vi "Auton Builder.vi"() -> ()   [LabVIEW 2018]
uses:
  Typedef/Robot Settings.ctl
  Typedef/Data Point.ctl
  Typedef/Robot Starting Position.ctl
  Typedef/Sequence Command.ctl
  Typedef/Plate Arrangement.ctl
  <vilib>/Utility/miscctls.llb/LVRowAndColumnTypeDef.ctl
panel:
  in  "Start Position Names":T1
  in  "Stop?":bool
  in  "Tab Control":enum32{"Builder", "Raw Sequence", "Settings"}(tab)
  in  "Start Position":T1
  in  "Reverse Path":bool
  in  "Data Points":T2[](array[typedef])=[{"X"=68.0, "Y"=162.0, "Theta"=0.0, "Speed %"=0.0, "Disabled?"=FALSE}]
  in  "Open":bool
  in  "Save":bool
  in  "Reset":bool
  in  "Send to Robot":bool
  in  "Simulate":bool
  in  "Name":string
  out "Field Half":cluster{dbl[], dbl[]}[](graph)=[{[48.5, 82.0, 82.0, 48.5, 48.5], [176.25, 176.25, 147.75, 147.75, 176.25]}, {[68.0], [162.0]}, {[68.0], [162.0]}, {[81.13940299900052], [156.48469503745656]}, {[54.86059700099948], [167.51530496254344]}]
  in  "Cancel":bool
  out "Location Names":string[](array[string])=["Center", "Left Level 1", "Right Level 1", "Left Level 2", "Right Level 2"]
  in  "Locations":cluster{"X":dbl, "Y":dbl}[](array[cluster])=[{"X"=68.0, "Y"=162.0}, {"X"=68.0, "Y"=212.0}, {"X"=68.0, "Y"=112.0}, {"X"=19.5, "Y"=212.0}, {"X"=19.5, "Y"=112.0}]
  in  "Path Folder":path=path "C:/Users/RoboChargers/Documents/LabVIEW Data/Deep-Space-2019/Auton/Paths"
  in  "Robot Settings":T3={"Width"=28.5, "Length"=33.5, "Center of Rotation"=19.5} caption="Robot Settings w/ Bumpers"
  # "LEFT"
  # "FAR"
  # "NEAR"
  # "RIGHT"
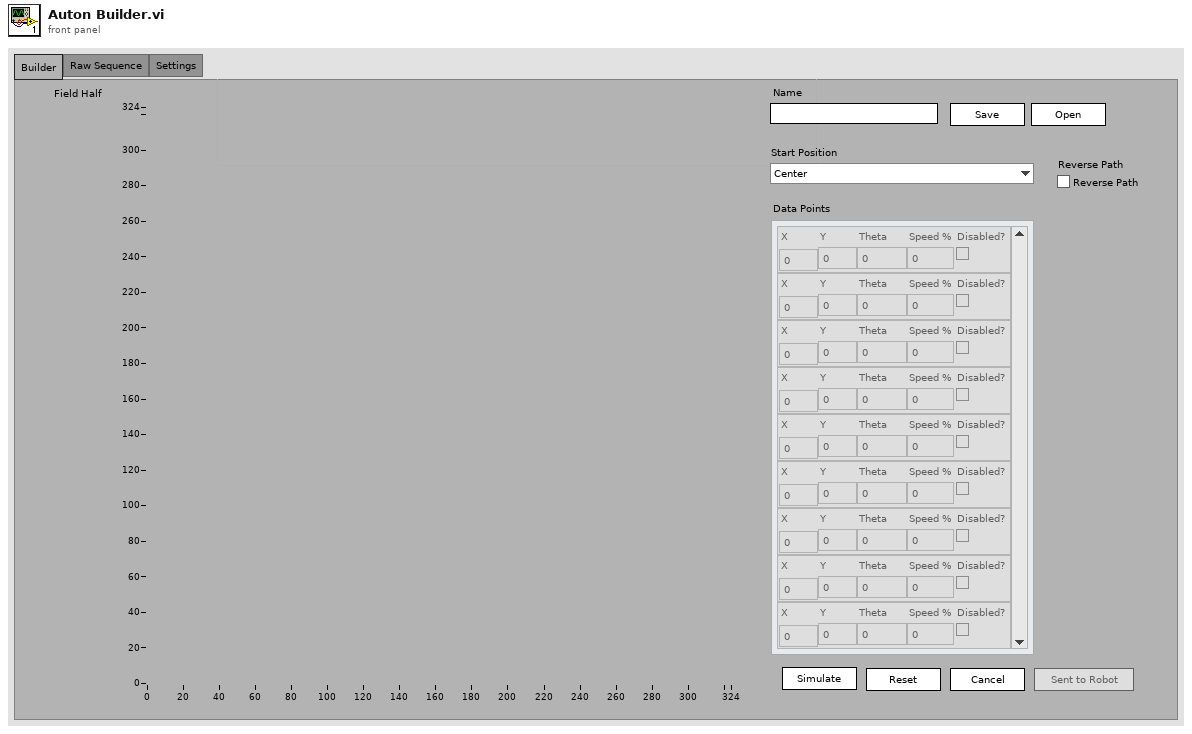
[diagram p1: front panel]
types:
  T1 = typedef "Robot Starting Position.ctl" = enum16{"Center", "Left Level 1", "Right Level 1", "Left Level 2", "Right Level 2"}
  T2 = typedef "Data Point.ctl" = cluster{"X":dbl, "Y":dbl, "Theta":dbl, "Speed %":dbl, "Disabled?":bool}
  T3 = typedef "Robot Settings.ctl" = cluster{"Width":dbl, "Length":dbl, "Center of Rotation":dbl}
  T4 = typedef "Sequence Command.ctl" = cluster{"Sequence Name":string, "Plate Arrangement":T5, "Command Name":string, "Data":variant, "Sequence Number":u32}
  T5 = typedef "Plate Arrangement.ctl" = cluster{"LR*":bool, "LL*":bool, "RL*":bool, "RR*":bool}
  T6 = typedef "LVRowAndColumnTypeDef.ctl" = cluster{"Row":i32, "Column":i32}
  T7 = cluster{"Field Half":cluster{dbl[], dbl[]}[], "Current Command":T4, "Robot Position":cluster{"x":dbl, "y":dbl}, "Theta":dbl, "y position":dbl, "Active Cell":T6, "Robot Index":i32, "Sequence OK?":bool, "Start Position":cluster{"x":dbl, "y":dbl}, "Field Selection":string, "Simulation Index":i32, "Sim Robot Index":i32, "Active Path":path, "Load Index":i32, "Graph Index":i32, "Data Points Index":i32, "Data Points":T2[], "Path Index":i32, "Path L Index":i32, "Path R Index":i32}
  T8 = typedef "LVPoint32TypeDef.ctl" = cluster{"Horizontal":i32, "Vertical":i32}
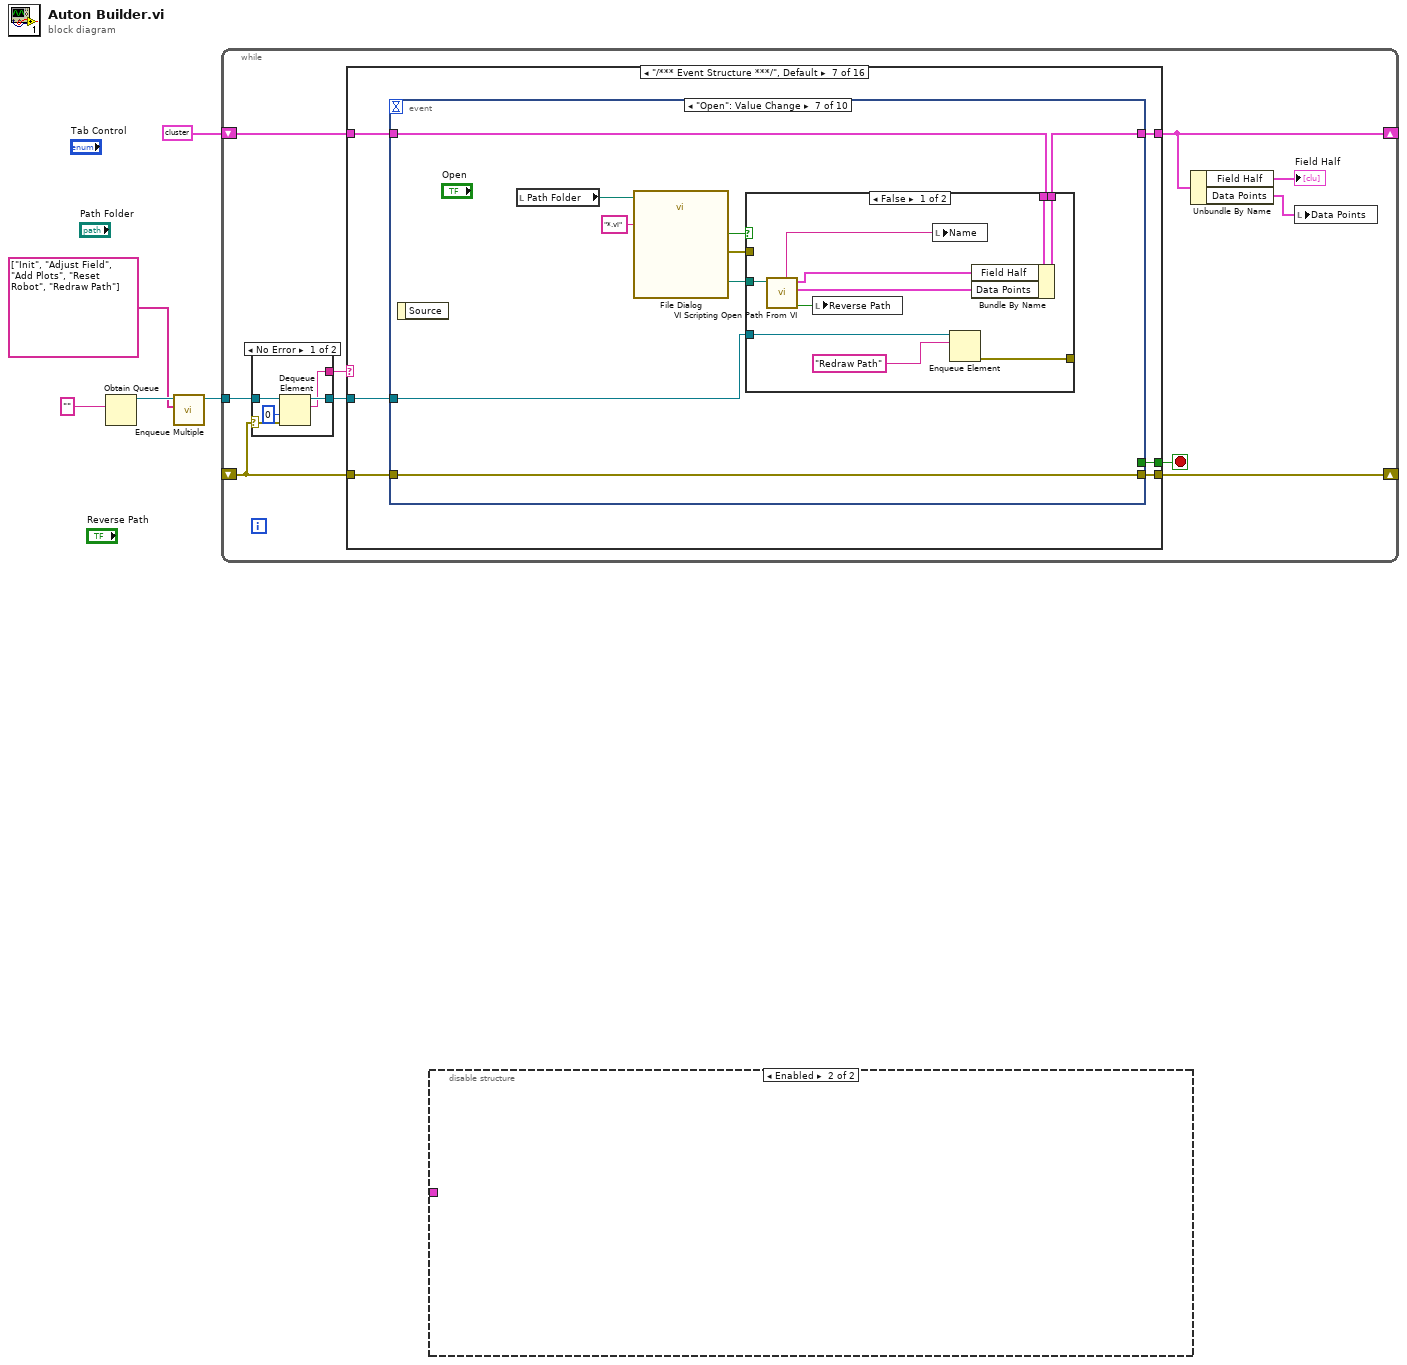
[diagram p0: block diagram]
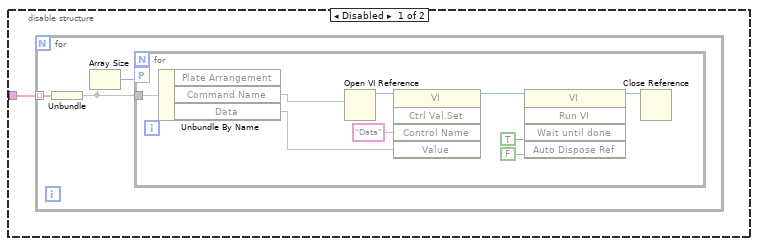
[diagram p2: hidden frame]
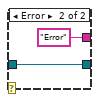
[diagram p3: hidden frame]
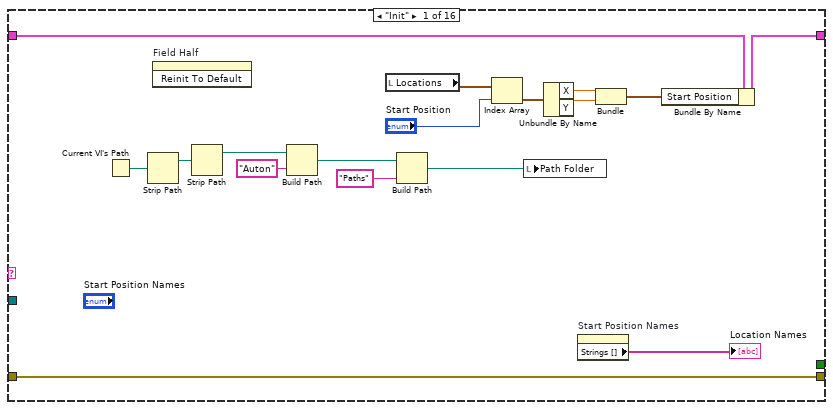
[diagram p4: hidden frame]
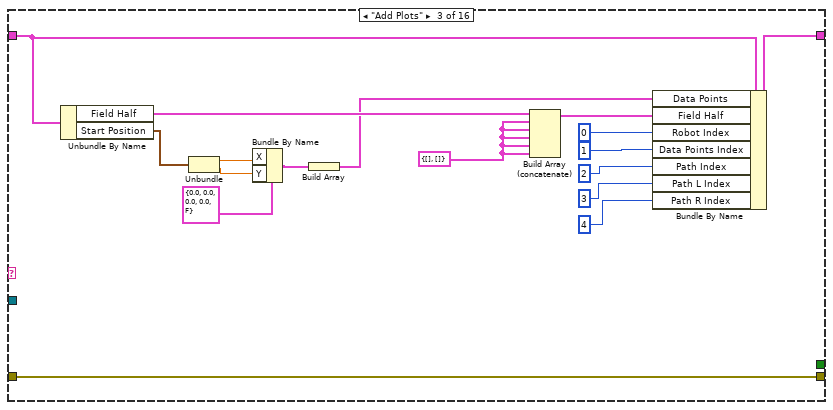
[diagram p6: hidden frame]
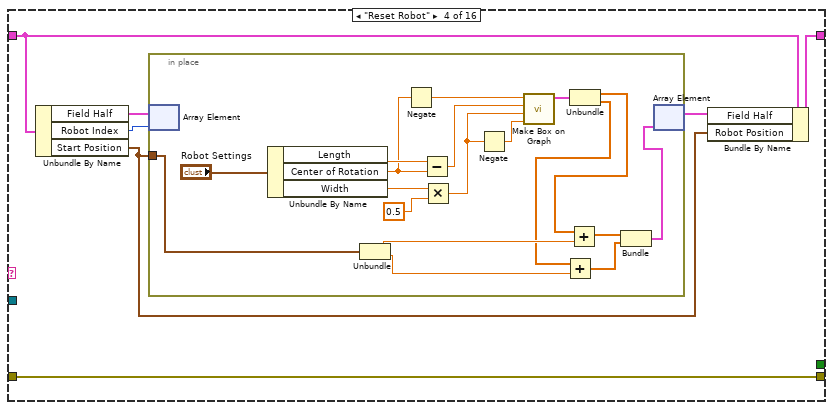
[diagram p7: hidden frame]
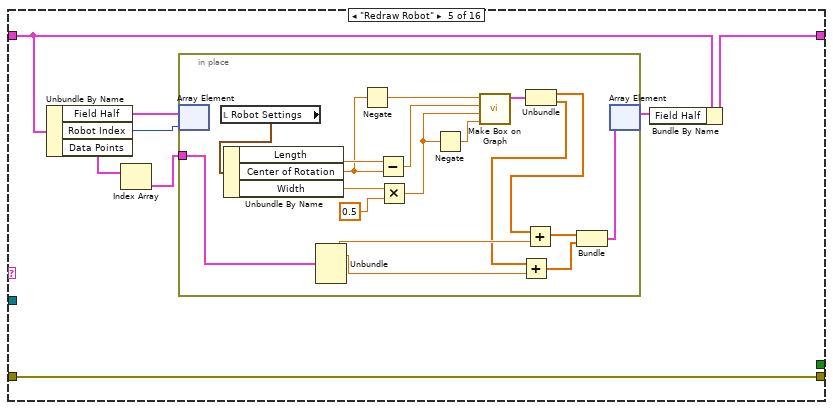
[diagram p8: hidden frame]
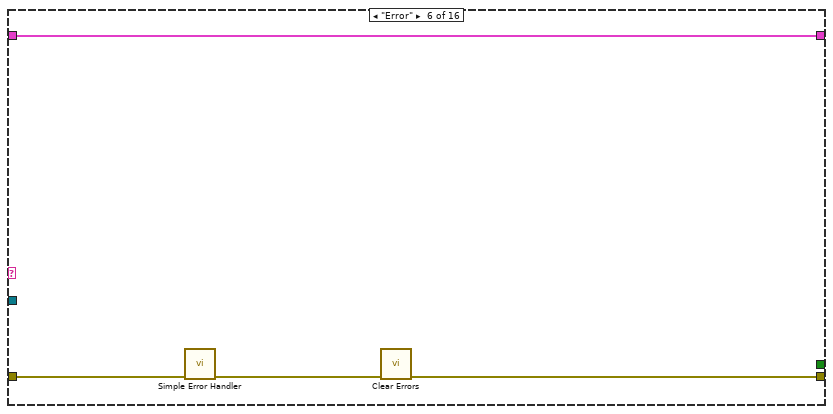
[diagram p9: hidden frame]
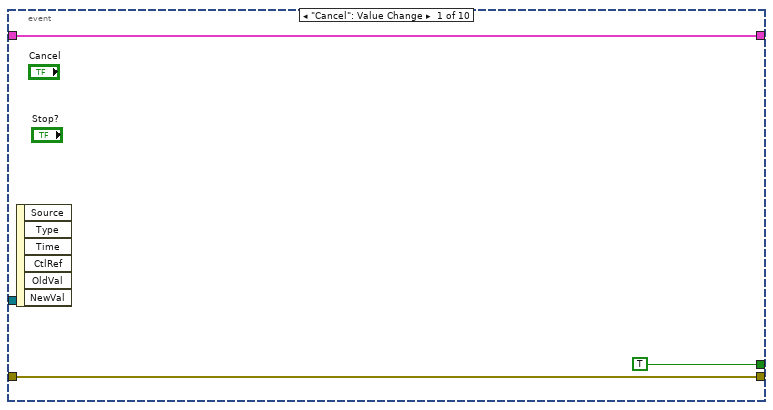
[diagram p10: hidden frame]
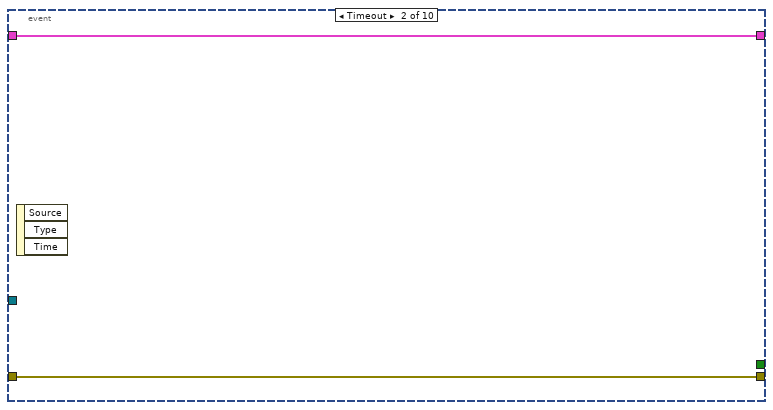
[diagram p11: hidden frame]
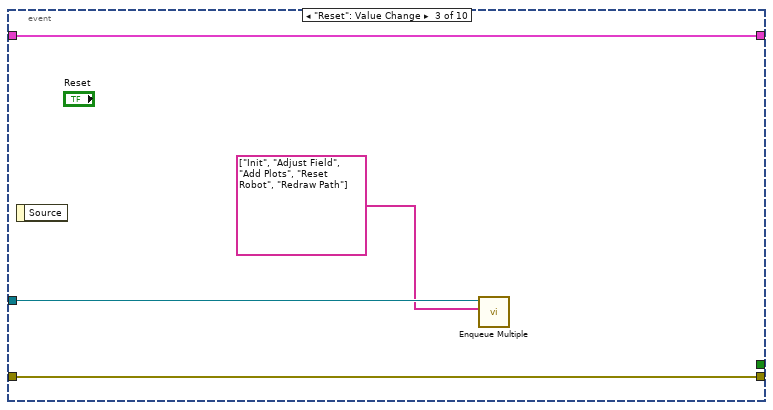
[diagram p12: hidden frame]
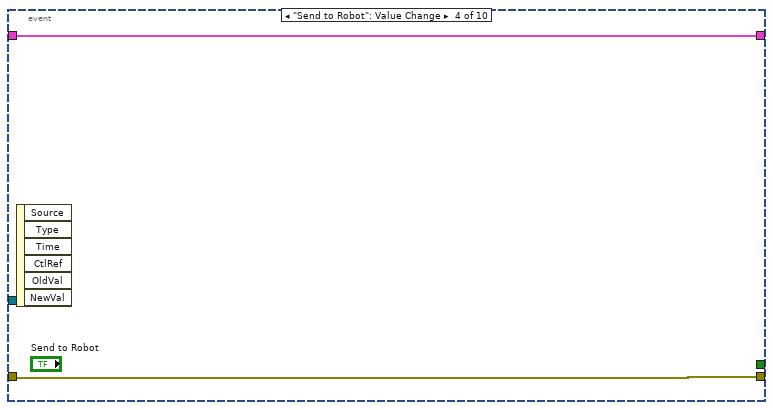
[diagram p13: hidden frame]
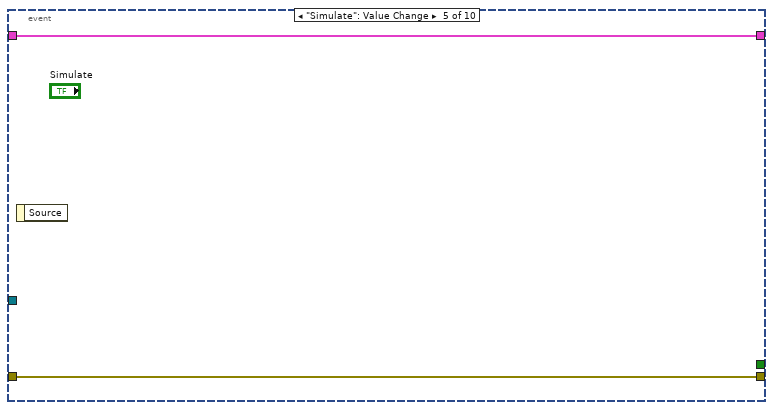
[diagram p14: hidden frame]
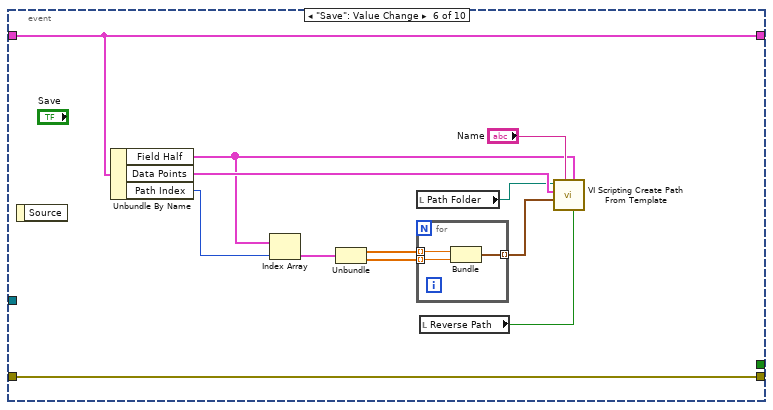
[diagram p15: hidden frame]
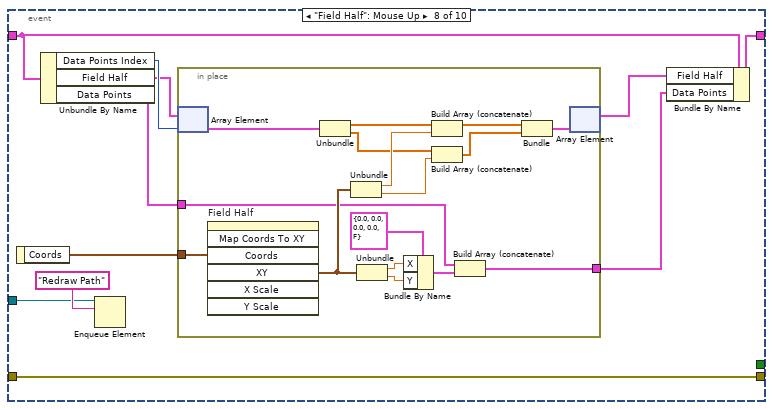
[diagram p17: hidden frame]
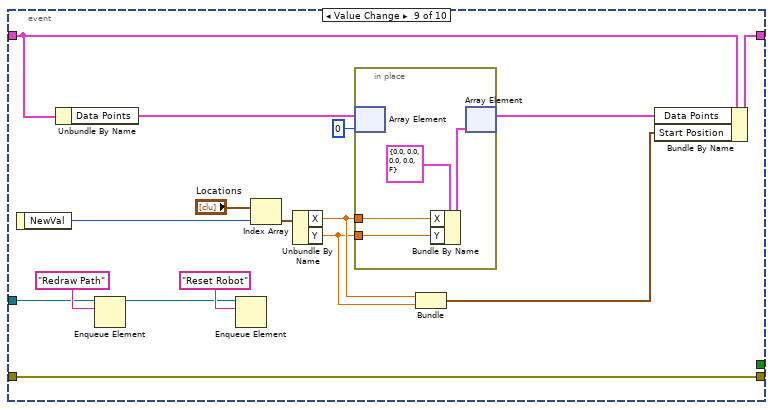
[diagram p18: hidden frame]
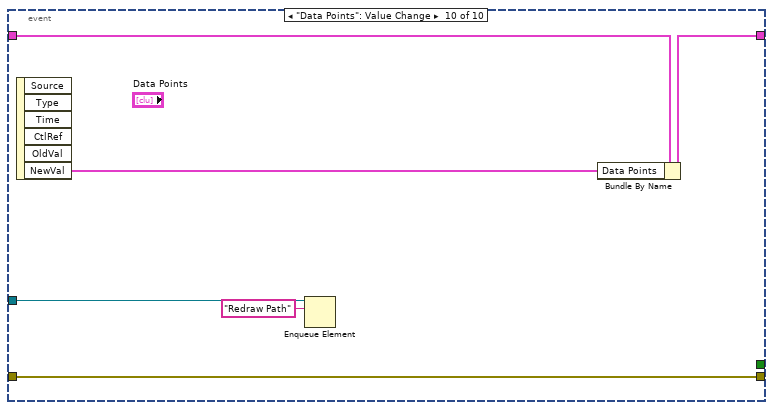
[diagram p19: hidden frame]
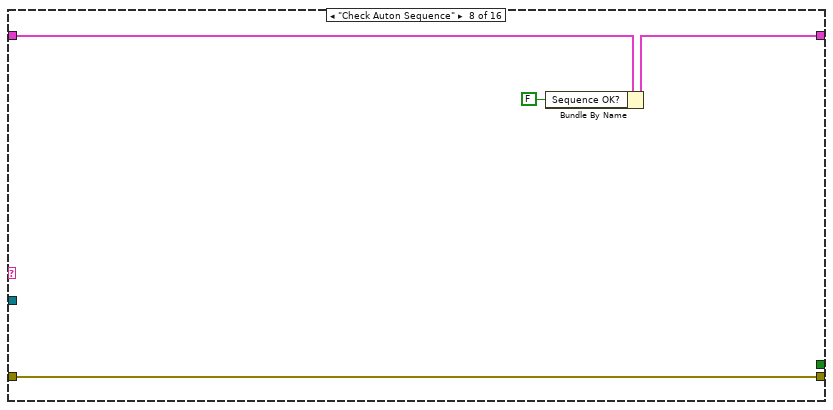
[diagram p20: hidden frame]
diagram:
  n1 = Obtain Queue(element data type="") -> (queue out=w4:refnum<queue>)  [unwired: 4 in, 2 out]
  n2 = call "Enqueue Multiple.vi"("Array"=string[] ["Init", "Adjust Field", "Add Plots", "Reset Robot", "Redraw Path"], "Queue in"=w4) -> ("Queue out"=w3:refnum<queue>)  [unwired: 8 in, 1 out]
  n3 = while {
    shift-right: [w9] -> _
    shift-left: T7 {"Field Half"=[], "Current Command"={"Sequence Name"="", "Plate Arrangement"={"LR*"=FALSE, "LL*"=FALSE, "RL*"=FALSE, "RR*"=FALSE}, "Command Name"="", "Data"=variant, "Sequence Number"=0}, "Robot Position"={"x"=0.0, "y"=0.0}, "Theta"=0.0, "y position"=0.0, "Active Cell"={"Row"=0, "Column"=0}, "Robot Index"=0, "Sequence OK?"=FALSE, "Start Position"={"x"=0.0, "y"=0.0}, "Field Selection"="", "Simulation Index"=0, "Sim Robot Index"=0, "Active Path"=path "", "Load Index"=0, "Graph Index"=0, "Data Points Index"=0, "Data Points"=[], "Path Index"=0, "Path L Index"=0, "Path R Index"=0} ("output cluster") -> [w15]
    shift-right: [w11] -> _
    shift-left: _ -> [w10]
    tunnel: w3 -> [w14]
    stop <- w7 stop-if-true
    n4 = case shown="No Error" w10 {
      selector: w10 -> [w18 _]
      tunnel: w14 -> [w20 w22]
      tunnel: [w19 w22] -> w13
      tunnel: [w17 "Error"] -> w12
      frame No Error {
        n5 = Dequeue Element(queue=w20, timeout in ms (-1)=0, error in (no error)=w18) -> (queue out=w19:refnum<queue>, element=w17:string)  [unwired: 2 out]
      }
      frame Error {
      }
    }
    n6 = case shown="\"/*** Event Structure ***/\", Default" w12 {
      tunnel: [_ _ _ _ _ _ w119 _ _ _ _ _ _ _ _ _] -> w7
      tunnel: w15 -> [w39 w40 w56 w64 w90 w113 w118 w223 w235 w250 w262 w278 w307 w312 w314 w316]
      tunnel: [w38 w40 w58 w65 w91 w113 w117 w222 w228 w246 w261 w276 w307 w310 w314 w316] -> w9
      tunnel: w13 -> [_ _ _ _ _ _ w116 _ _ _ _ w269 _ _ _ _]
      tunnel: [w37 w41 w54 w63 w89 w112 w114 w224 w226 w244 w263 w279 w306 w311 w313 w315] -> w11
      tunnel: w10 -> [w37 w41 w54 w63 w89 w111 w115 w224 w226 w244 w263 w279 w306 w311 w313 w315]
      frame "Init" {
        n7 = Current VI's Path() -> (path=w36:path)
        n8 = Strip Path(path=w36) -> (stripped path=w35:path)  [unwired: 1 out]
        n9 = invoke on="Field Half" class="XYGraph (strict)" method="Reinit To Default"() -> ()  [unwired: 3 in, 3 out]
        n10 = Strip Path(path=w35) -> (stripped path=w34:path)  [unwired: 1 out]
        n11 = Build Path(base path=w34, name or relative path="Auton") -> (appended path=w32:path)
        n12 = local read "Locations"() -> (w24:cluster{"X":dbl, "Y":dbl}[])
        n13 = Build Path(base path=w32, name or relative path="Paths") -> (appended path=w30:path)
        n14 = Index Array(array=w24, index="Start Position") -> (element=w28:cluster{"X":dbl, "Y":dbl})
        n15 = local write "Path Folder"(w30) -> ()
        n16 = Unbundle By Name(w28) -> ("X"=w27:dbl, "Y"=w26:dbl)
        n17 = property on="Start Position Names" class="Enum (strict)"() -> ("Strings []"=→"Location Names":string[])  [unwired: 2 in, 2 out]
        n18 = Bundle("X"=w27, "Y"=w26) -> (w25:cluster{"X":dbl, "Y":dbl})  [unwired: 1 in]
        n19 = Bundle By Name(cluster=w39, "Start Position"=w25) -> (w38:T7)
      }
      frame "Adjust Field" {
      }
      frame "Add Plots" {
        w47 = cluster{dbl[], dbl[]} {[], []} ("element")
        n20 = Unbundle By Name(w56) -> ("Field Half"=w55:cluster{dbl[], dbl[]}[], "Start Position"=w48:cluster{"x":dbl, "y":dbl})
        n21 = Unbundle(w48) -> ("x"=w45:dbl, "y"=w44:dbl)
        n22 = Bundle By Name(cluster=T2 {"X"=0.0, "Y"=0.0, "Theta"=0.0, "Speed %"=0.0, "Disabled?"=FALSE} ("Cluster"), "X"=w45, "Y"=w44) -> (w43:T2)
        n23 = Build Array(w43) -> (w42:T2[])
        n24 = Build Array (concatenate)(w55, w47, w47, w47, w47, w47) -> (w57:cluster{dbl[], dbl[]}[])
        n25 = Bundle By Name(cluster=w56, "Data Points"=w42, "Field Half"=w57, "Robot Index"=0, "Data Points Index"=1 ("Spline Index"), "Path Index"=2 ("Spline Index"), "Path L Index"=3 ("Spline Index"), "Path R Index"=4 ("Spline Index")) -> (w58:T7)
      }
      frame "Reset Robot" {
        n26 = Unbundle By Name(w64) -> ("Field Half"=w62:cluster{dbl[], dbl[]}[], "Robot Index"=w61:i32, "Start Position"=w59:cluster{"x":dbl, "y":dbl})
        n27 = in-place {
          in-place-border: w59 -> [w83]
          n28 = in-place-array #1(w62, w61) -> ()  [unwired: 1 out]
          n29 = Unbundle By Name("Robot Settings") -> ("Length"=w73:dbl, "Center of Rotation"=w72:dbl, "Width"=w77:dbl)
          n30 = Unbundle(w83) -> ("x"=w82:dbl, "y"=w81:dbl)
          n31 = Negate(x=w72) -> (-x=w74:dbl)
          n32 = Subtract(x=w73, y=w72) -> (x-y=w71:dbl)
          n33 = Multiply(x=w77, y=0.5 ("x")) -> (x*y=w76:dbl)
          n34 = Negate(x=w76) -> (-x=w75:dbl)
          n35 = call "Make Box on Graph.vi"("Y2"=w75, "Y1"=w76, "X2"=w71, "X1"=w74) -> ("Output Graph"=w69:cluster{dbl[], dbl[]})  [unwired: 7 in]
          n36 = Unbundle(w69) -> (w68:dbl[], w67:dbl[])
          n37 = Add(x=w67, y=w81) -> (x+y=w80:dbl[])
          n38 = Add(x=w68, y=w82) -> (x+y=w79:dbl[])
          n39 = Bundle(w79, w80) -> (w66:cluster{dbl[], dbl[]})  [unwired: 1 in]
          n40 = in-place-array #1(w66) -> (w60:cluster{dbl[], dbl[]}[])  [unwired: 1 out]
        }
        n41 = Bundle By Name(cluster=w64, "Field Half"=w60, "Robot Position"=w59) -> (w65:T7)
      }
      frame "Redraw Robot" {
        n42 = Unbundle By Name(w90) -> ("Field Half"=w88:cluster{dbl[], dbl[]}[], "Robot Index"=w87:i32, "Data Points"=w86:T2[])
        n43 = Index Array(array=w86) -> (element=w85:T2)  [unwired: 1 in]
        n44 = in-place {
          in-place-border: w85 -> [w109]
          n45 = in-place-array #2(w88, w87) -> ()  [unwired: 1 out]
          n46 = local read "Robot Settings"() -> (w93:T3)
          n47 = Unbundle By Name(w93) -> ("Length"=w100:dbl, "Center of Rotation"=w99:dbl, "Width"=w104:dbl)
          n48 = Unbundle(w109) -> ("X"=w108:dbl, "Y"=w107:dbl)  [unwired: 3 out]
          n49 = Negate(x=w99) -> (-x=w101:dbl)
          n50 = Subtract(x=w100, y=w99) -> (x-y=w98:dbl)
          n51 = Multiply(x=w104, y=0.5 ("x")) -> (x*y=w103:dbl)
          n52 = Negate(x=w103) -> (-x=w102:dbl)
          n53 = call "Make Box on Graph.vi"("Y2"=w102, "Y1"=w103, "X2"=w98, "X1"=w101) -> ("Output Graph"=w96:cluster{dbl[], dbl[]})  [unwired: 7 in]
          n54 = Unbundle(w96) -> (w95:dbl[], w94:dbl[])
          n55 = Add(x=w94, y=w107) -> (x+y=w106:dbl[])
          n56 = Add(x=w95, y=w108) -> (x+y=w105:dbl[])
          n57 = Bundle(w105, w106) -> (w92:cluster{dbl[], dbl[]})  [unwired: 1 in]
          n58 = in-place-array #2(w92) -> (w84:cluster{dbl[], dbl[]}[])  [unwired: 1 out]
        }
        n59 = Bundle By Name(cluster=w90, "Field Half"=w84) -> (w91:T7)
      }
      frame "Error" {
        n60 = call <vilib>:"Simple Error Handler.vi"("error in (no error)"=w111) -> ("error out"=w110:errorcluster)  [unwired: 4 in, 4 out]
        n61 = call <vilib>:"Clear Errors.vi"("error in (no error)"=w110) -> ("error out"=w112:errorcluster)  [unwired: 5 in, 1 out]
      }
      frame "/*** Event Structure ***/", Default {
        n62 = event shown="[6] \"Open\": Value Change" {
          selector: _ -> [_ _ _ _ _ _ _ _ _ _]
          dyn-events: _ -> [_ _ _ _ _ _ _ _ _ _]
          timeout: _ -> [_ _ _ _ _ _ _ _ _ _]
          tunnel: [TRUE _ _ _ _ _ _ _ _ _] -> w119
          tunnel: w118 -> [w121 w124 w128 w130 w132 w144 w150 w174 w209 w219]
          tunnel: [w121 w124 w128 w130 w132 w144 w149 w172 w208 w218] -> w117
          tunnel: w116 -> [_ _ w127 _ _ _ w148 w168 w206 w216]
          tunnel: w115 -> [w120 w123 w126 w129 w131 w140 w156 w178 w210 w220]
          tunnel: [w120 w123 w126 w129 w131 w140 w156 w178 w210 w220] -> w114
          event "Cancel": Value Change {
            n63 = event-data() -> ()  [unwired: 1 in, 6 out]
          }
          event Timeout {
            n64 = event-data() -> ()  [unwired: 1 in, 3 out]
          }
          event "Reset": Value Change {
            n65 = event-data() -> ()  [unwired: 1 in, 1 out]
            n66 = call "Enqueue Multiple.vi"("Array"=string[] ["Init", "Adjust Field", "Add Plots", "Reset Robot", "Redraw Path"], "Queue in"=w127) -> ()  [unwired: 8 in, 2 out]
          }
          event "Send to Robot": Value Change {
            n67 = event-data() -> ()  [unwired: 1 in, 6 out]
          }
          event "Simulate": Value Change {
            n68 = event-data() -> ()  [unwired: 1 in, 1 out]
          }
          event "Save": Value Change {
            n69 = event-data() -> ()  [unwired: 1 in, 1 out]
            n70 = Unbundle By Name(w144) -> ("Field Half"=w138:cluster{dbl[], dbl[]}[], "Data Points"=w142:T2[], "Path Index"=w137:i32)
            n71 = Index Array(array=w138, index=w137) -> (element=w136:cluster{dbl[], dbl[]})
            n72 = Unbundle(w136) -> (w134:dbl[], w135:dbl[])
            n73 = local read "Path Folder"() -> (w139:path)
            n74 = for {
              tunnel: [w147] -> w141 mode=indexing
              tunnel: w135 -> [w146] mode=indexing
              tunnel: w134 -> [w145] mode=indexing
              n75 = Bundle("x"=w145, "y"=w146) -> (w147:cluster{"x":dbl, "y":dbl})  [unwired: 1 in]
            }
            n76 = local read "Reverse Path"() -> (w133:bool)
            n77 = call "VI Scripting Create Path From Template.vi"("Reverse Path?"=w133, "Graph"=w138, "Name"="Name", "path"=w141, "Data Points"=w142, "base path"=w139) -> ()  [unwired: 6 in]
          }
          event "Open": Value Change {
            n78 = event-data() -> ()  [unwired: 1 in, 1 out]
            n79 = local read "Path Folder"() -> (w154:path)
            n80 = call "File Dialog"("start path"=w154, "pattern (all files)"="*.vi") -> ("selected path"=w155:path, "cancelled"=w153:bool, "error out"=w152:errorcluster)  [unwired: 10 in, 1 out]
            n81 = case shown="False" w153 {
              tunnel: w155 -> [w166 _]
              tunnel: w150 -> [w165 w167]
              tunnel: [w163 w167] -> w149
              tunnel: w148 -> [w160 _]
              tunnel: w152 -> [_ _]
              tunnel: [w157 _] -> _
              frame False {
                n82 = call "VI Scripting Open Path From VI.vi"("Path"=w166) -> ("Reverse Path?"=w164:bool, "Data Points"=w161:T2[], "Graph"=w162:cluster{dbl[], dbl[]}[], "Name"=w158:string)  [unwired: 6 in, 1 out]
                n83 = local write "Reverse Path"(w164) -> ()
                n84 = local write "Name"(w158) -> ()
                n85 = Enqueue Element(queue=w160, element="Redraw Path") -> (error out=w157:errorcluster)  [unwired: 2 in, 2 out]
                n86 = Bundle By Name(cluster=w165, "Field Half"=w162, "Data Points"=w161) -> (w163:T7)
              }
              frame True {
              }
            }
          }
          event "Field Half": Mouse Up {
            n87 = event-data() -> ("Coords"=w177:T8)  [unwired: 1 in]
            n88 = Unbundle By Name(w174) -> ("Data Points Index"=w176:i32, "Field Half"=w175:cluster{dbl[], dbl[]}[], "Data Points"=w170:T2[])
            n89 = Enqueue Element(queue=w168, element="Redraw Path") -> ()  [unwired: 2 in, 3 out]
            n90 = in-place {
              in-place-border: w177 -> [w186]
              in-place-border: [w180] -> w171
              in-place-border: w170 -> [w179]
              n91 = in-place-array #3(w175, w176) -> (w194:cluster{dbl[], dbl[]})
              n92 = invoke on="Field Half" class="XYGraph (strict)" method="Map Coords To XY"("Coords"=w186) -> ("XY"=w184:cluster{"X":dbl, "Y":dbl})  [unwired: 6 in, 6 out]
              n93 = Unbundle(w194) -> (w192:dbl[], w191:dbl[])
              n94 = Unbundle(w184) -> ("X"=w193:dbl, "Y"=w190:dbl)
              n95 = Unbundle(w184) -> ("X"=w183:dbl, "Y"=w182:dbl)
              n96 = Bundle By Name(cluster=T2 {"X"=0.0, "Y"=0.0, "Theta"=0.0, "Speed %"=0.0, "Disabled?"=FALSE} ("Cluster"), "X"=w183, "Y"=w182) -> (w185:T2)
              n97 = Build Array (concatenate)(w192, w193) -> (w189:dbl[])
              n98 = Build Array (concatenate)(w191, w190) -> (w188:dbl[])
              n99 = Build Array (concatenate)(w179, w185) -> (w180:T2[])
              n100 = Bundle(w189, w188) -> (w187:cluster{dbl[], dbl[]})  [unwired: 1 in]
              n101 = in-place-array #3(w187) -> (w173:cluster{dbl[], dbl[]}[])  [unwired: 1 out]
            }
            n102 = Bundle By Name(cluster=w174, "Field Half"=w173, "Data Points"=w171) -> (w172:T7)
          }
          event Value Change {
            n103 = event-data() -> ("NewVal"=w200:T1)  [unwired: 1 in]
            n104 = Unbundle By Name(w209) -> ("Data Points"=w204:T2[])
            n105 = Enqueue Element(queue=w206, element="Redraw Path") -> (queue out=w198:refnum<queue>)  [unwired: 2 in, 2 out]
            n106 = Enqueue Element(queue=w198, element="Reset Robot") -> ()  [unwired: 2 in, 3 out]
            n107 = Index Array(array="Locations", index=w200) -> (element=w201:cluster{"X":dbl, "Y":dbl})
            n108 = Unbundle By Name(w201) -> ("X"=w197:dbl, "Y"=w196:dbl)
            n109 = in-place {
              in-place-border: w197 -> [w212]
              in-place-border: w196 -> [w211]
              n110 = in-place-array #4(w204, 0) -> ()  [unwired: 1 out]
              n111 = Bundle By Name(cluster=T2 {"X"=0.0, "Y"=0.0, "Theta"=0.0, "Speed %"=0.0, "Disabled?"=FALSE} ("element"), "X"=w212, "Y"=w211) -> (w214:T2)
              n112 = in-place-array #4(w214) -> (w205:T2[])  [unwired: 1 out]
            }
            n113 = Bundle("X"=w197, "Y"=w196) -> (w195:cluster{"X":dbl, "Y":dbl})  [unwired: 1 in]
            n114 = Bundle By Name(cluster=w209, "Data Points"=w205, "Start Position"=w195) -> (w208:T7)
          }
          event "Data Points": Value Change {
            n115 = event-data() -> ("NewVal"=w217:T2[])  [unwired: 1 in, 5 out]
            n116 = Enqueue Element(queue=w216, element="Redraw Path") -> ()  [unwired: 2 in, 3 out]
            n117 = Bundle By Name(cluster=w219, "Data Points"=w217) -> (w218:T7)
          }
        }
      }
      frame "Check Auton Sequence" {
        n118 = Bundle By Name(cluster=w223, "Sequence OK?"=FALSE) -> (w222:T7)
      }
      frame "Handle Graph Delete" {
        n119 = Unbundle By Name(w235) -> ("Field Half"=w229:cluster{dbl[], dbl[]}[], "Current Command"=w234:T4)
        n120 = Unbundle By Name(w234) -> ("Data"=w233:variant)
        n121 = Get Variant Attribute(Variant=w233, name="_graphIndex", default value (empty Variant)=0) -> (found=w225:bool, value=w231:i32)  [unwired: 1 in, 2 out]
        n122 = case shown="True" w225 {
          tunnel: w231 -> [_ w239]
          tunnel: w229 -> [w236 w238]
          tunnel: [w236 w237] -> w227
          frame False {
          }
          frame True {
            n123 = in-place {
              n124 = in-place-array #5(w238, w239) -> ()  [unwired: 1 out]
              n125 = in-place-array #5(cluster{dbl[], dbl[]} {[], []} ("element")) -> (w237:cluster{dbl[], dbl[]}[])  [unwired: 1 out]
            }
          }
        }
        n126 = Bundle By Name(cluster=w235, "Field Half"=w227) -> (w228:T7)
      }
      frame "Add Robot Plot" {
        n127 = Unbundle By Name(w250) -> ("Field Half"=w243:cluster{dbl[], dbl[]}[], "Current Command.Data"=w249:variant)
        n128 = Index Array(array=w243) -> (element=w241:cluster{dbl[], dbl[]})  [unwired: 1 in]
        n129 = Get Variant Attribute(Variant=w249, name="_graphPlot") -> (found=w247:bool, value=w242:variant)  [unwired: 2 in, 2 out]
        n130 = case shown="True" w247 {
          tunnel: [w251 w256] -> w245
          tunnel: w243 -> [w251 w255]
          tunnel: w242 -> [_ w254]
          tunnel: w241 -> [_ w253]
          frame False {
          }
          frame True {
            n131 = Variant To Data(type=w253, Variant=w254) -> (data=w252:cluster{dbl[], dbl[]})  [unwired: 1 in, 1 out]
            n132 = Build Array (concatenate)(w255, w252) -> (w256:cluster{dbl[], dbl[]}[])
          }
        }
        n133 = Bundle By Name(cluster=w250, "Field Half"=w245) -> (w246:T7)
      }
      frame "Update Graph Index" {
        n134 = Unbundle By Name(w262) -> ("Field Half"=w260:cluster{dbl[], dbl[]}[], "Graph Index"=w259:i32, "Current Command.Data"=w258:variant)
        n135 = in-place {
          in-place-border: w258 -> [w266]
          n136 = in-place-array #6(w260, w259) -> ()  [unwired: 1 out]
          n137 = Get Variant Attribute(Variant=w266, name="_graphPlot", default value (empty Variant)=cluster{dbl[], dbl[]} {[], []} ("value")) -> (value=w264:cluster{dbl[], dbl[]})  [unwired: 1 in, 3 out]
          n138 = in-place-array #6(w264) -> (w257:cluster{dbl[], dbl[]}[])  [unwired: 1 out]
        }
        n139 = Bundle By Name(cluster=w262, "Field Half"=w257) -> (w261:T7)
      }
      frame "Redraw Path" {
        n140 = Unbundle By Name(w278) -> ("Data Points"=w274:T2[], "Field Half"=w277:cluster{dbl[], dbl[]}[], "Data Points Index"=w270:i32, "Path Index"=w271:i32, "Path L Index"=w272:i32, "Path R Index"=w273:i32)
        n141 = Enqueue Element(queue=w269, element="Redraw Robot") -> ()  [unwired: 2 in, 3 out]
        n142 = in-place {
          in-place-border: w274 -> [w288]
          n143 = in-place-array #7(w277, w270, w271, w272, w273) -> ()  [unwired: 4 out]
          n144 = for {
            tunnel: [w305] -> w293 mode=indexing
            tunnel: w288 -> [w304] mode=indexing
            tunnel: [w303] -> w284 mode=indexing
            tunnel: [w302] -> w283 mode=indexing
            n145 = Unbundle(w304) -> ("X"=w303:dbl, "Y"=w302:dbl)  [unwired: 3 out]
            n146 = Bundle("X"=w303, "Y"=w302) -> (w305:cluster{"X":dbl, "Y":dbl})  [unwired: 1 in]
          }
          n147 = local read "Robot Settings"() -> (w281:T3)
          n148 = call "Path Inject Points.vi"("Distance"=1.0, "Path"=w293) -> ("Path out"=w298:cluster{dbl, dbl}[])  [unwired: 9 in]
          n149 = Bundle(w284, w283) -> (w282:cluster{dbl[], dbl[]})  [unwired: 1 in]
          n150 = Unbundle By Name(w281) -> ("Width"=w280:dbl)
          n151 = call "Path Smoother.vi"("tolerance"=0.001, "B"=0.95, "A"=0.05, "Path"=w298) -> ("SmoothPath"=w292:cluster{dbl, dbl}[])  [unwired: 7 in]
          n152 = for {
            tunnel: w292 -> [w301] mode=indexing
            tunnel: [w300] -> w290 mode=indexing
            tunnel: [w299] -> w291 mode=indexing
            n153 = Unbundle(w301) -> (w300:dbl, w299:dbl)
          }
          n154 = Bundle(w290, w291) -> (w285:cluster{dbl[], dbl[]})  [unwired: 1 in]
          n155 = call "Path to Wheel Path.vi"("Wheelbase (in)"=w280, "waypoints"=w285) -> ("out"=w289:cluster{dbl[], dbl[]}[])  [unwired: 9 in]
          n156 = Index Array(array=w289) -> (element #1=w286:cluster{dbl[], dbl[]}, element #2=w287:cluster{dbl[], dbl[]})  [unwired: 2 in]
          n157 = in-place-array #7(w282, w285, w286, w287) -> (w275:cluster{dbl[], dbl[]}[])  [unwired: 4 out]
        }
        n158 = Bundle By Name(cluster=w278, "Field Half"=w275) -> (w276:T7)
      }
      frame "/**** Simulation Functions ****/" {
      }
      frame "Simulation Init" {
        n159 = Bundle By Name(cluster=w312, "Simulation Index"=0, "Sim Robot Index"=0) -> (w310:T7)
      }
      frame "Select Field String" {
      }
      frame "/**** File Operations ****/" {
      }
    }
    n160 = Unbundle By Name(w9) -> ("Field Half"=→"Field Half":cluster{dbl[], dbl[]}[], "Data Points"=w6:T2[])
    n161 = local write "Data Points"(w6) -> ()
  }
  n162 = disable-structure shown="Enabled" {
    disable-tunnel: _ -> [w317 _]
    frame Disabled {
      n163 = for {
        tunnel: w317 -> [w320] mode=indexing
        n164 = Unbundle(w320) -> ("Sequence Array"=w318)
        n165 = Array Size(array=w318) -> (size(s)=w319:i32)
        n166 = for {
          tunnel: w318 -> [w329]
          workers-P: w319 -> [_]
          n167 = Unbundle By Name(w329) -> ("Command Name"=w325, "Data"=w327)  [unwired: 1 out]
          n168 = Open VI Reference(vi path=w325) -> (vi reference=w328:refnum<vi>)  [unwired: 5 in, 1 out]
          n169 = invoke class="VI" method="Ctrl Val.Set"(reference=w328, "Control Name"="Data", "Value"=w327) -> (reference out=w324:refnum<vi>)  [unwired: 2 in, 4 out]
          n170 = invoke class="VI" method="Run VI"(reference=w324, "Wait until done"=TRUE ("Wait Until Done"), "Auto Dispose Ref"=FALSE ("Auto Dispose Reference")) -> (reference out=w323:refnum<vi>)  [unwired: 2 in, 4 out]
          n171 = Close Reference(reference=w323) -> ()  [unwired: 1 in, 1 out]
        }
      }
    }
    frame Enabled {
    }
  }
